vi "GenerateUntriggeredStimulus.vi"(8 "error in (no error)":errorcluster, 11 "HeadTailContinuousGWN in":refnum<class "HeadTailContinuousGWN.lvclass">) -> (0 "error out":errorcluster, 2 "UntriggeredStimulusOut (uW/mm^2)":sgl[][](array[numeric]), 3 "HeadTailContinuousGWN out":refnum<class "HeadTailContinuousGWN.lvclass">)   [LabVIEW 2019, in "HeadTailContinuousGWN.lvclass"]
uses:
  HeadTailContinuousGWN.lvclass
  C:/Users/Mochi/Dropbox/LeiferShaevitz/Github/ProjectAPI/LabviewVIs/StimulusObject.lvclass
  StimulusObject.lvclass/StimulusObject.ctl
  HeadTailContinuousGWN.lvclass/HeadTailContinuousGWN.ctl
  ParametersGlobal.vi
  <vilib>/ptbypt/Signal Generation.llb/Gaussian White Noise PtByPt.vi
  StimulusObject.lvclass
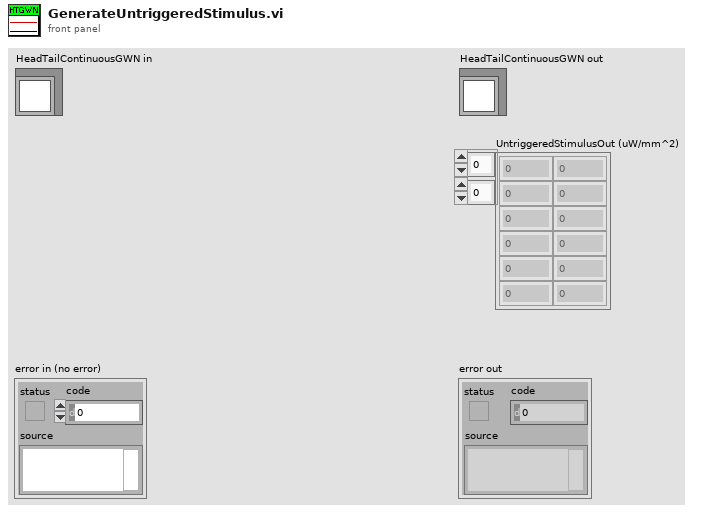
[diagram p1: front panel]
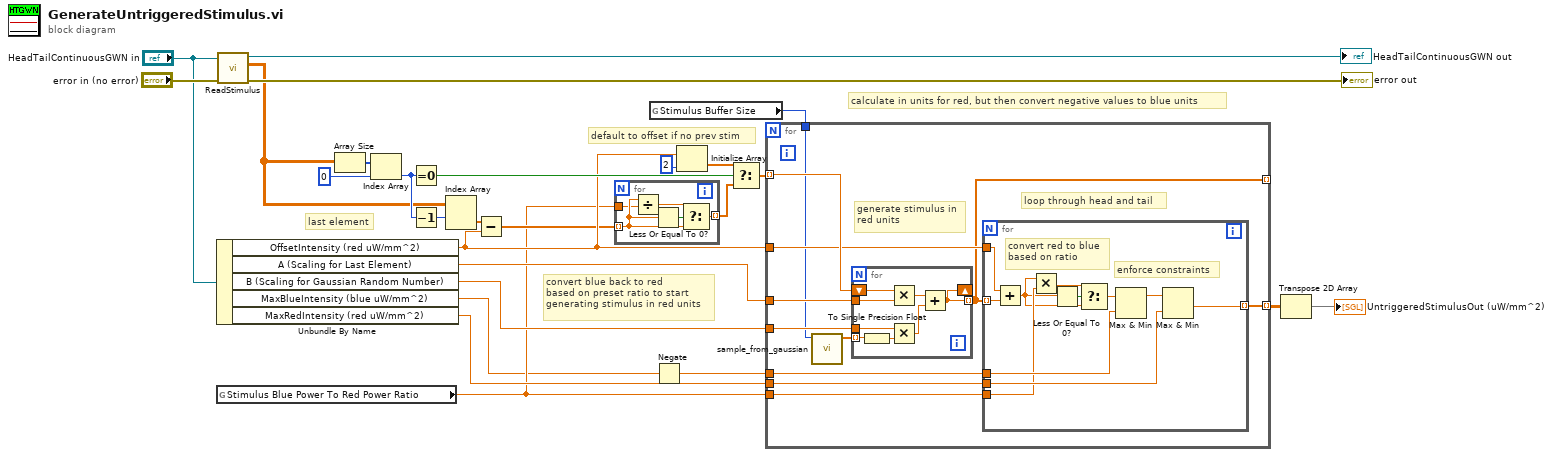
[diagram p0: block diagram]
diagram:
  # "convert blue back to red\nbased on preset ratio to start\ngenerating stimulus in red units"
  # "calculate in units for red, but then convert negative values to blue units"
  # "default to offset if no prev stim"
  # "last element"
  n1 = Unbundle By Name("HeadTailContinuousGWN in") -> ("OffsetIntensity (red uW/mm^2)"=w8:sgl, "A (Scaling for Last Element)"=w18:sgl, "B (Scaling for Gaussian Random Number)"=w17:sgl, "MaxBlueIntensity (blue uW/mm^2)"=w2:sgl, "MaxRedIntensity (red uW/mm^2)"=w16:sgl)
  n2 = global read "ParametersGlobal.vi" "Stimulus Blue Power To Red Power Ratio"() -> (w3:sgl)
  n3 = call "ReadStimulus.vi"("error in (no error)"="error in (no error)", "StimulusObject in"="HeadTailContinuousGWN in") -> ("error out"=→"error out":errorcluster, "StimulusOut"=w4:sgl[][], "StimulusObject out"=→"HeadTailContinuousGWN out":refnum<class "HeadTailContinuousGWN.lvclass">)  [unwired: 7 in]
  n4 = Array Size(array=w4) -> (size(s)=w26:i32[])
  n5 = Index Array(array=w26, index=0) -> (element=w21:i32)
  n6 = Equal To 0?(x=w21) -> (x = 0?=w24:bool)
  n7 = Decrement(x=w21) -> (x-1=w20:i32)
  n8 = Index Array(array=w4, index (row)=w20) -> (element=w22:sgl[])  [unwired: 1 in]
  n9 = Subtract(x=w22, y=w8) -> (x-y=w6:sgl[])
  n10 = for {
    tunnel: w6 -> [w28] mode=indexing
    tunnel: [w30] -> w5 mode=indexing
    tunnel: w3 -> [w27]
    n11 = Divide(x=w28, y=w27) -> (x/y=w29:sgl)
    n12 = Less Or Equal To 0?(x=w28) -> (x <= 0?=w31:bool)
    n13 = Select(t=w29, s=w31, f=w28) -> (s? t:f=w30:sgl)
  }
  n14 = global read "ParametersGlobal.vi" "Stimulus Buffer Size"() -> (w10:i32)
  n15 = Negate(x=w2) -> (-x=w1:sgl)
  n16 = Initialize Array(w8, 2 ("dimension size")) -> (w9:sgl[])
  n17 = Select(t=w9, s=w24, f=w5) -> (s? t:f=w23:sgl[])
  n18 = for {
    tunnel: w23 -> [w42] mode=indexing
    tunnel: w18 -> [w41]
    tunnel: w17 -> [w40]
    tunnel: [w38] -> w19 mode=indexing
    tunnel: w8 -> [w37]
    tunnel: w1 -> [w36]
    tunnel: w16 -> [w35]
    tunnel: w10 -> [w34]
    tunnel: w3 -> [w33]
    tunnel: [w32] -> _ mode=indexing
    # "generate stimulus in\nred units"
    # "loop through head and tail"
    n19 = call "sample_from_gaussian.vi"("Samples"=w34) -> ("Output"=w39:dbl[])  [unwired: 10 in]
    n20 = for {
      shift-right: [w54] -> _
      shift-left: w42 -> [w60]
      tunnel: w41 -> [w61]
      tunnel: w40 -> [w57]
      tunnel: w39 -> [w59] mode=indexing
      tunnel: [w54] -> w32 mode=indexing
      n21 = To Single Precision Float(number=w59) -> (single precision float=w58:sgl)
      n22 = Multiply(x=w60, y=w61) -> (x*y=w55:sgl)
      n23 = Multiply(x=w57, y=w58) -> (x*y=w56:sgl)
      n24 = Add(x=w55, y=w56) -> (x+y=w54:sgl)
    }
    n25 = for {
      tunnel: w32 -> [w51] mode=indexing
      tunnel: [w52] -> w38 mode=indexing
      tunnel: w37 -> [w50]
      tunnel: w36 -> [w49]
      tunnel: w35 -> [w48]
      tunnel: w33 -> [w44]
      # "convert red to blue\nbased on ratio"
      # "enforce constraints"
      n26 = Add(x=w50, y=w51) -> (x+y=w43:sgl)
      n27 = Multiply(x=w43, y=w44) -> (x*y=w46:sgl)
      n28 = Less Or Equal To 0?(x=w43) -> (x <= 0?=w47:bool)
      n29 = Select(t=w46, s=w47, f=w43) -> (s? t:f=w45:sgl)
      n30 = Max & Min(x=w45, y=w49) -> (max(x,y)=w53:sgl)  [unwired: 1 out]
      n31 = Max & Min(x=w53, y=w48) -> (min(x,y)=w52:sgl)  [unwired: 1 out]
    }
  }
  n32 = Transpose 2D Array(2D array=w19) -> (transposed array=→"UntriggeredStimulusOut (uW/mm^2)":sgl[][])
